vi "ExtractFromDat.vi"() -> ()   [LabVIEW 2014]
uses:
  <vilib>/Utility/file.llb/Write To Spreadsheet File (DBL).vi
panel:
  in  "FileName":string
  in  "stop":bool
  out "Numeric":i32
  out "error out":errorcluster
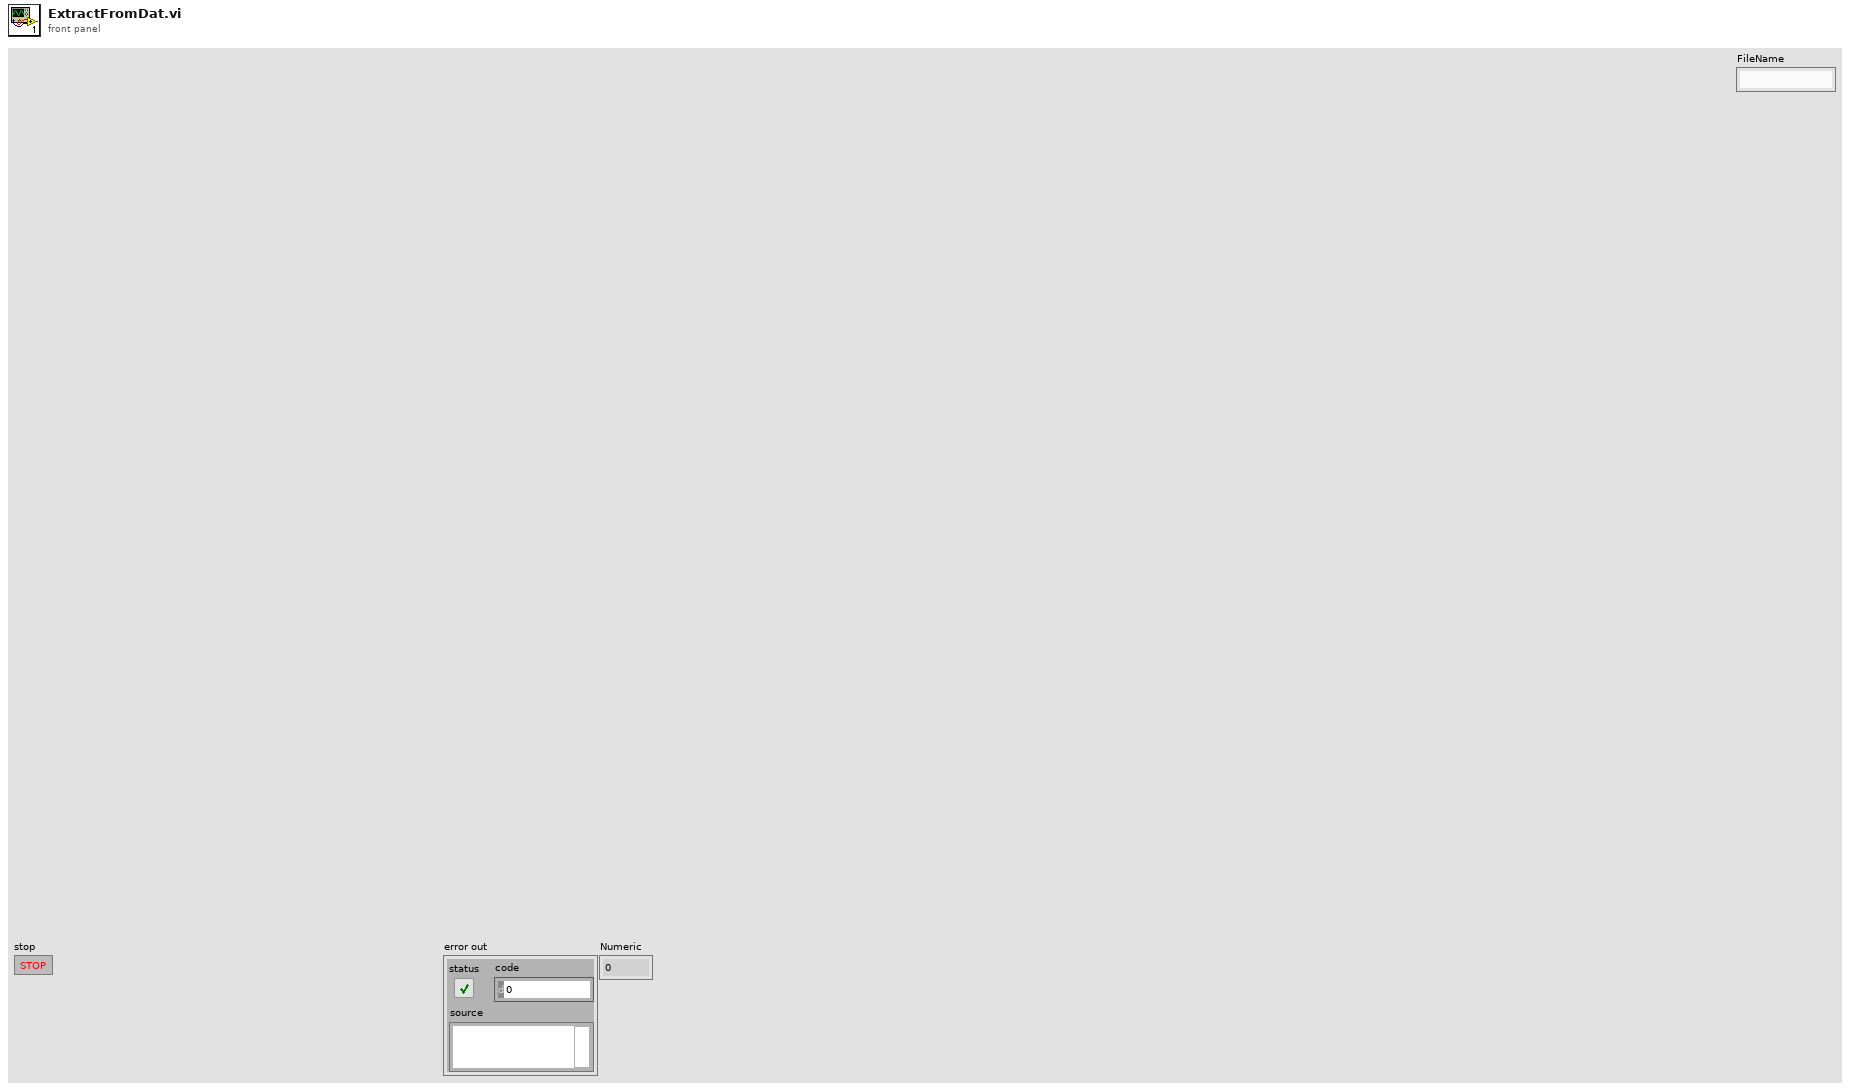
[diagram p1: front panel]
types:
  T1 = cluster{"gpsTimeUTC":i64, "cT":dbl, "EKF VelN":sgl, "EKF VelE":sgl, "EKF VelD":sgl, "EKF PosN":sgl, "EKF PosE":sgl, "EKF PosD":sgl, "EKF Roll":sgl, "EKF Pitch":sgl, "EKF Yaw":sgl, "EKF Lat":dbl, "EKF Lon":dbl, "EKF Alt":sgl, "CMP VelN":sgl, "CMP VelE":sgl, "CMP VelD":sgl, "CMP PosN":sgl, "CMP PosE":sgl, "CMP PosD":sgl, "CMP Roll":sgl, "CMP Pitch":sgl, "CMP Yaw":sgl, "CMP Lat":dbl, "CMP Lon":dbl, "CMP Alt":sgl, "GPS Lat":dbl, "GPS Lon":dbl, "GPS Alt":sgl, "GPS VelN":sgl, "GPS VelE":sgl, "GPS VelD":sgl, "AccelX":sgl, "AccelY":sgl, "AccelZ":sgl, "GyroX":sgl, "GyroY":sgl, "GyroZ":sgl, "MagX":sgl, "MagY":sgl, "MagZ":sgl, "piAlpha":sgl, "piPfwd":u16, "piP45":u16, "ardAlpha":sgl, "ardPfwd":u16, "ardP45":u16, "Alpha":sgl, "Beta":sgl}
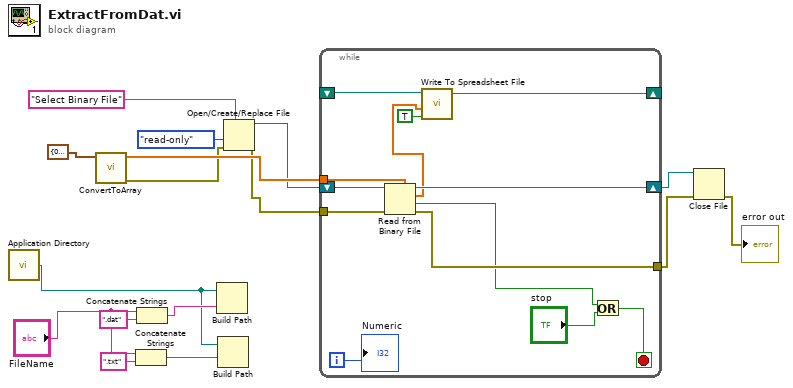
[diagram p0: block diagram]
diagram:
  n1 = call <vilib>:"Application Directory.vi"() -> ("Application Directory"=w1:path)
  n2 = call "ConvertToArray.vi"("Cluster"=T1 {"gpsTimeUTC"=0, "cT"=0.0, "EKF VelN"=0.0, "EKF VelE"=0.0, "EKF VelD"=0.0, "EKF PosN"=0.0, "EKF PosE"=0.0, "EKF PosD"=0.0, "EKF Roll"=0.0, "EKF Pitch"=0.0, "EKF Yaw"=0.0, "EKF Lat"=0.0, "EKF Lon"=0.0, "EKF Alt"=0.0, "CMP VelN"=0.0, "CMP VelE"=0.0, "CMP VelD"=0.0, "CMP PosN"=0.0, "CMP PosE"=0.0, "CMP PosD"=0.0, "CMP Roll"=0.0, "CMP Pitch"=0.0, "CMP Yaw"=0.0, "CMP Lat"=0.0, "CMP Lon"=0.0, "CMP Alt"=0.0, "GPS Lat"=0.0, "GPS Lon"=0.0, "GPS Alt"=0.0, "GPS VelN"=0.0, "GPS VelE"=0.0, "GPS VelD"=0.0, "AccelX"=0.0, "AccelY"=0.0, "AccelZ"=0.0, "GyroX"=0.0, "GyroY"=0.0, "GyroZ"=0.0, "MagX"=0.0, "MagY"=0.0, "MagZ"=0.0, "piAlpha"=0.0, "piPfwd"=0, "piP45"=0, "ardAlpha"=0.0, "ardPfwd"=0, "ardP45"=0, "Alpha"=0.0, "Beta"=0.0}) -> ("error out"=w9:errorcluster, "Array"=w15:dbl[])  [unwired: 9 in]
  n3 = Concatenate Strings("FileName", ".txt" ("string")) -> (w3:string)
  n4 = Concatenate Strings("FileName", ".dat" ("string")) -> (w2:string)
  n5 = Build Path(base path=w1, name or relative path=w2) -> ()  [unwired: 1 out]
  n6 = Build Path(base path=w1, name or relative path=w3) -> ()  [unwired: 1 out]
  n7 = Open/Create/Replace File(error in=w9, prompt="Select Binary File", access (0:read/write)=enum16{"read/write", "read-only", "write-only"}."read-only") -> (refnum out=w14:refnum<file>, error out=w10:errorcluster)  [unwired: 3 in, 1 out]
  n8 = while {
    tunnel: w15 -> [w29]
    shift-right: [w26] -> _
    shift-left: _ -> [w25]
    tunnel: w10 -> [w23]
    tunnel: [w22] -> w12
    shift-right: [w28] -> w13
    shift-left: w14 -> [w27]
    i -> [w21]
    stop <- w18 stop-if-true
    n9 = Read from Binary File(5:w29, 8:w23, 11:w27) -> (0:w22:errorcluster, 1:w17:bool, 2:w20:dbl[], 3:w28:refnum<file>)  [unwired: 3 in]
    n10 = call-poly <vilib>:"Write To Spreadsheet File.vi"("append to file? (new file:F)"=TRUE, "1D data"=w20, "file path (dialog if empty)"=w25) -> ("new file path (Not A Path if cancelled)"=w26:path)  [unwired: 5 in]
    n11 = Or(x=w17, y="stop") -> (x .or. y?=w18:bool)
    "Numeric" <- w21
  }
  n12 = Close File(refnum=w13, error in=w12) -> (error out=→"error out":errorcluster)  [unwired: 1 out]
